vi "set_url.vi"(8 "error in (no error)":errorcluster, 10 "Array in":string[](array[string])=["tree", "DecisionTreeClassifier", "fit"], 11 "VI in":refnum<vi>) -> (0 "error out":errorcluster, 3 "VI out":refnum<vi>)   [LabVIEW 2020]
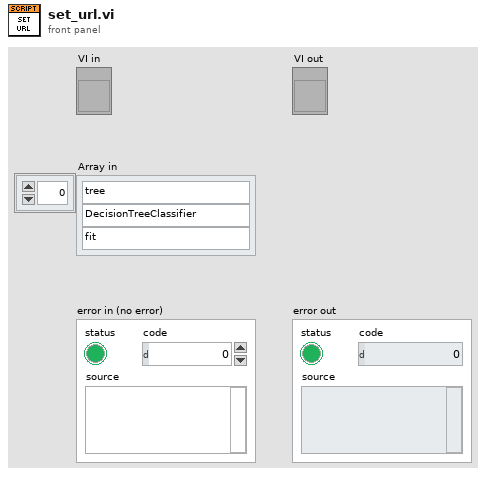
[diagram p1: front panel]
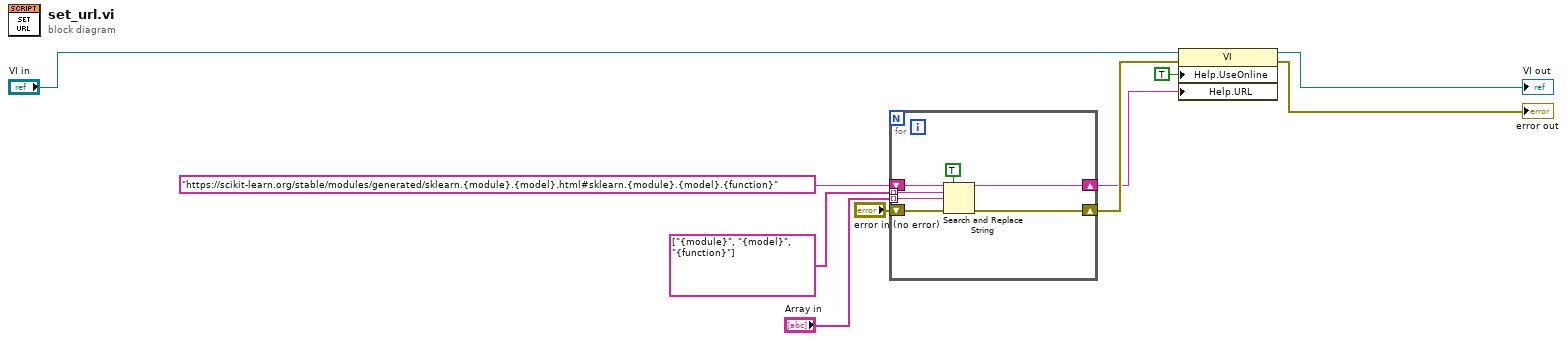
[diagram p0: block diagram]
diagram:
  n1 = for {
    tunnel: string[] ["{module}", "{model}", "{function}"] -> [w16] mode=indexing
    shift-right: [w14] -> w6
    shift-left: "https://scikit-learn.org/stable/modules/generated/sklearn.{module}.{model}.html#sklearn.{module}.{model}.{function}" -> [w17]
    tunnel: "Array in" -> [w15] mode=indexing
    shift-right: [w13] -> w8
    shift-left: "error in (no error)" -> [w12]
    n2 = Search and Replace String(replace all?=TRUE ("replace all? (F)"), input string=w17, search string=w16, replace string=w15, error in=w12) -> (result string=w14:string, error out=w13:errorcluster)  [unwired: 3 in, 2 out]
  }
  n3 = property class="VI"(reference="VI in", error in=w8, "Help.UseOnline"=TRUE ("Help:Use Web URL"), "Help.URL"=w6) -> (reference out=→"VI out":refnum<vi>, error out=→"error out":errorcluster)
